vi "Dispatch Transfer Group.vi"(6 "Iteration":u64, 7 "command":T1, 8 "error in (no error)":errorcluster, 9 "Transfer Group ID":i32, 10 "Plugin ID":i32, 11 "Dispatcher Interface in":refnum<class "Dispatcher Interface.lvclass">) -> (0 "error out":errorcluster, 3 "Dispatcher Interface out":refnum<class "Dispatcher Interface.lvclass">)   [LabVIEW 2017, in "DSF Core.lvlib" / "Dispatcher Interface.lvclass"]
uses:
  Interfaces/Dispatcher/Dispatcher Interface.lvclass
  C:/Git/DSF/Data Sharing Framework/Source/Core/Engine/Classes/Interfaces/Interface/Interface.lvclass
  Interfaces/Dispatcher/Command.ctl
  Interfaces/Dispatcher/Rx Parameters.ctl
  Interfaces/Interface/Interface.lvclass/Interface.ctl
  Interfaces/Dispatcher/Write.vi
  Interfaces/Dispatcher/Write Dispatcher Command.vi
  Interfaces/Interface/Send Command.vi
  Interfaces/Interface/Write RT FIFO.vi
  Interfaces/Interface/Errors.vi
  Interfaces/Dispatcher/Command Timeout.vi
  VIs/VI Name.vi
  Interfaces/Dispatcher/Class Name.vi
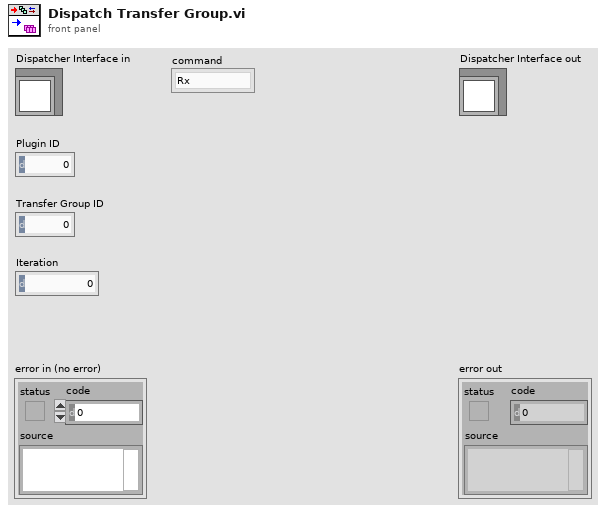
[diagram p1: front panel]
types:
  T1 = typedef "DSF Core.lvlib/Dispatcher Interface.lvclass/Command.ctl" = enum8{"Rx", "Tx", "Set Inline Buffer", "Shutdown"}
  T2 = typedef "DSF Core.lvlib/Dispatcher Interface.lvclass/Rx Parameters.ctl" = cluster{"Plugin ID":i32, "Transfer Group ID":i32, "Iteration":u64}
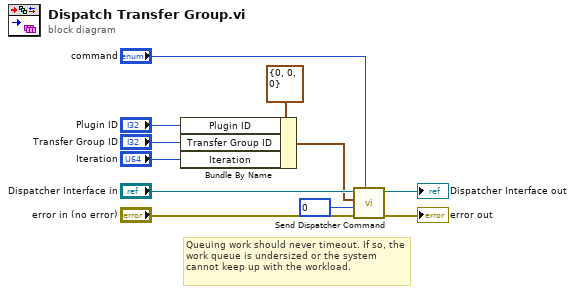
[diagram p0: block diagram]
diagram:
  # "Queuing work should never timeout. If so, the work queue is undersized or the system cannot keep up with the workload."
  n1 = Bundle By Name(cluster=T2 {"Plugin ID"=0, "Transfer Group ID"=0, "Iteration"=0} ("Rx Parameters"), "Plugin ID"="Plugin ID", "Transfer Group ID"="Transfer Group ID", "Iteration"="Iteration") -> (w6:T2)
  n2 = call "Send Dispatcher Command.vi"("Command"="command", "error in (no error)"="error in (no error)", "timeout in ms (0)"=0, "Rx Parameters"=w6, "Dispatcher Interface in"="Dispatcher Interface in") -> ("error out"=→"error out":errorcluster, "Dispatcher Interface out"=→"Dispatcher Interface out":refnum<class "Dispatcher Interface.lvclass">)  [unwired: 5 in]
